vi "Calibra.vi"() -> (1 "SurtOk?":bool)   [LabVIEW 2017]
uses:
  <vilib>/registry/registry.llb/Registry RtKey.ctl
  <vilib>/registry/registry.llb/Registry View.ctl
  <vilib>/registry/registry.llb/Write Registry Value Simple STR.vi
panel:
  in  "Nom Sensor Temperatura":string
  in  "error in (no error)":errorcluster
  in  "Cancel":bool
  in  "OK Button":bool
  out "error out":errorcluster
  in  "Pendent Temp_1":dbl
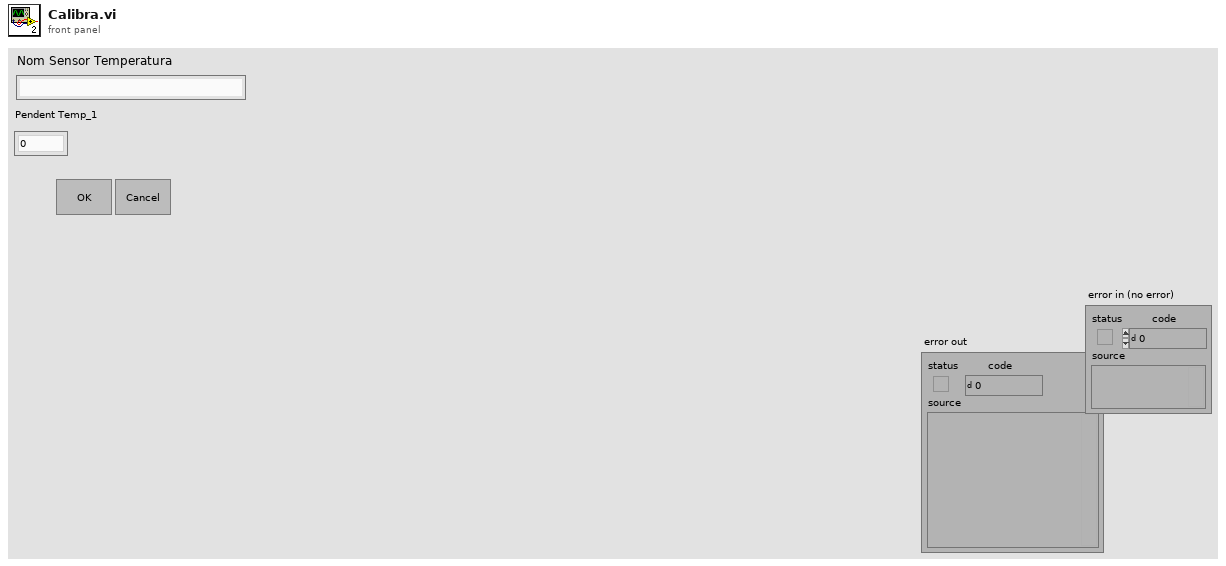
[diagram p1: front panel]
types:
  T1 = typedef "Registry RtKey.ctl" = enum32{"HKEY_CLASSES_ROOT", "HKEY_CURRENT_USER", "HKEY_LOCAL_MACHINE", "HKEY_USERS", "HKEY_PERFORMANCE_DATA", "HKEY_CURRENT_CONFIG", "HKEY_DYN_DATA"}
  T2 = typedef "Registry View.ctl" = u16
  T3 = typedef "Registry refnum.ctl" = refnum<k1>
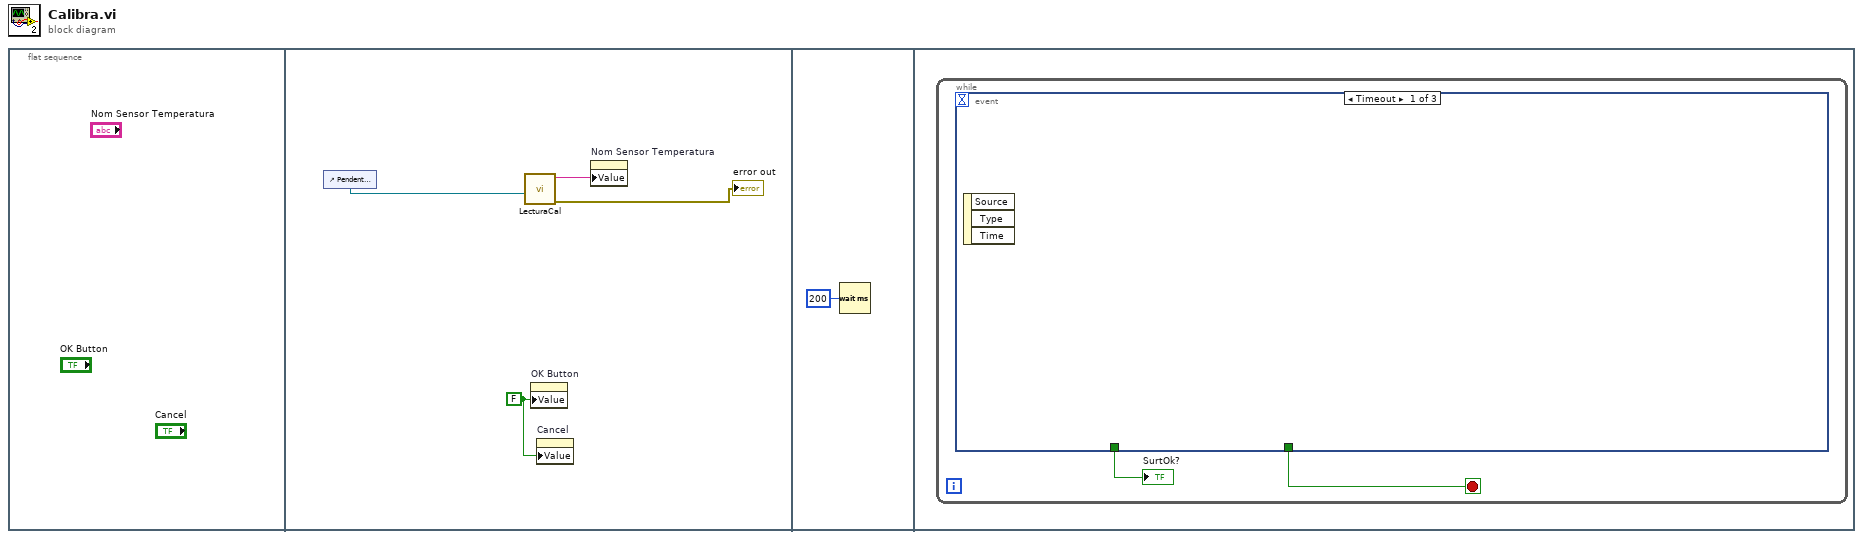
[diagram p0: block diagram]
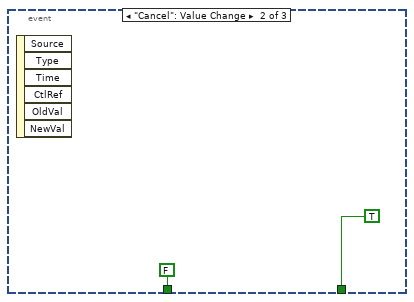
[diagram p2: hidden frame]
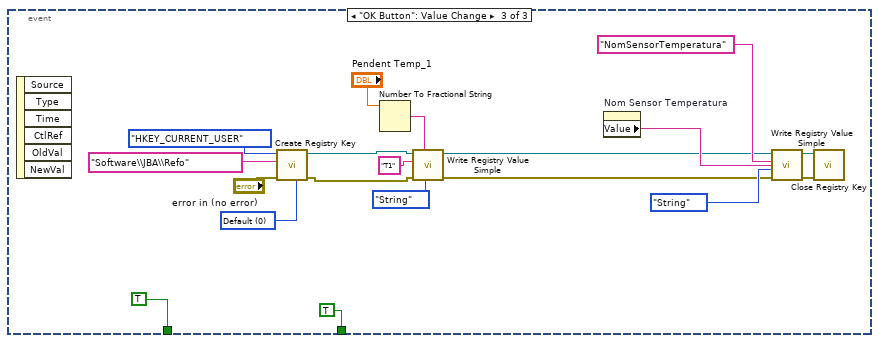
[diagram p3: hidden frame]
diagram:
  n1 = flat-sequence {
    frame #0 {
    }
    frame #1 {
      w2 = FALSE ("OK Button")
      n2 = control-ref of="Pendent Temp_1"() -> (w4:refnum<vi>)
      n3 = call "LecturaCal.vi"("T1"=w4) -> ("error out"=→"error out":errorcluster, "Nom Sensor Temperatura"=w1:string)  [unwired: 9 in]
      n4 = property on="OK Button" class="Bool (strict)"("Value"=w2) -> ()  [unwired: 2 in, 2 out]
      n5 = property on="Cancel" class="Bool (strict)"("Value"=w2) -> ()  [unwired: 2 in, 2 out]
      n6 = property on="Nom Sensor Temperatura" class="Str"("Value"=w1) -> ()  [unwired: 2 in, 2 out]
    }
    frame #2 {
      n7 = Wait (ms)(milliseconds to wait=u32 200) -> ()  [unwired: 1 out]
    }
    frame #3 {
      n8 = while {
        stop <- w7 stop-if-true
        n9 = event shown="[0] Timeout" {
          selector: _ -> [_ _ _]
          dyn-events: _ -> [_ _ _]
          timeout: _ -> [_ _ _]
          tunnel: [_ TRUE TRUE ("Ok?")] -> w7
          tunnel: [_ FALSE TRUE] -> w6
          event Timeout {
            n10 = event-data() -> ()  [unwired: 1 in, 3 out]
          }
          event "Cancel": Value Change {
            n11 = event-data() -> ()  [unwired: 1 in, 6 out]
          }
          event "OK Button": Value Change {
            w25 = T2 0 items=["Default"=0, "KEY_WOW64_64KEY"=8, "KEY_WOW64_32KEY"=9] ("registry view")
            n12 = event-data() -> ()  [unwired: 1 in, 6 out]
            n13 = call <vilib>:"Create Registry Key.vi"("registry view"=w25, "error in (no error)"="error in (no error)", "subkey"="Software\\JBA\\Refo", "root key (HKEY_LOCAL_MACHINE)"=Registry_RtKey."HKEY_CURRENT_USER") -> ("error out"=w13:errorcluster, "refnum out"=w14:T3)  [unwired: 5 in, 1 out]
            n14 = Number To Fractional String(number="Pendent Temp_1") -> (F-format string=w21:string)  [unwired: 3 in]
            n15 = call-poly <vilib>:"Write Registry Value Simple.vi"("String/Binary data"=w21, "error in (no error)"=w13, "simple data type"=enum16{"String", "Binary", "DWORD"}."String", "value"="T1", "refnum"=w14) -> ("error out"=w10:errorcluster, "refnum out"=w11:T3)  [unwired: 3 in]
            n16 = property on="Nom Sensor Temperatura" class="Str"() -> ("Value"=w16:string)  [unwired: 2 in, 2 out]
            n17 = call-poly <vilib>:"Write Registry Value Simple.vi"("String/Binary data"=w16, "error in (no error)"=w10, "simple data type"=enum16{"String", "Binary", "DWORD"}."String", "value"="NomSensorTemperatura", "refnum"=w11) -> ("error out"=w17:errorcluster, "refnum out"=w18:T3)  [unwired: 3 in]
            n18 = call <vilib>:"Close Registry Key.vi"("error in (no error)"=w17, "refnum"=w18) -> ()  [unwired: 5 in, 1 out]
          }
        }
        "SurtOk?" <- w6
      }
    }
  }
